vi "Balancing Controller.vi"(0 "Error In":errorcluster, 1 "steering indicator flag":i16, 5 "Trajectory In":refnum<data-value>, 6 "Balance In":refnum<data-value>, 9 "State Estimate In":refnum<data-value>, 10 "t":i32, 11 "Measurement In":refnum<data-value>, 12 "Indoor (RollRef)":bool=TRUE, 13 "Configuration":T1={"Accelerometer Bias"={"X (m/s)"=0.0, "Y (m/s)"=0.0, "Z (m/s)"=0.0}, "Gyroscope Bias"={"X (m/s)"=0.0, "Y (m/s)"=0.0, "Z (m/s)"=0.0}, "Steering Motor Gear Ratio"=611.0, "Steering Pully Gear Ratio"=1.0, "Steering Encoder CPR"=500.0, "Steering Motor Max RPM"=4000.0, "Wheelbase (m)"=1.12, "Fork Angle (rad)"=1.3, "Balancing Controller"={"Kp (/s)"=1.0, "Kd (1)"=1.0}, "Max Allowed Steering Angle (rad)"=0.7, "Task Periods"={"Emergency Stop (us)"=10000, "IMU (us)"=10000, "Steering Motor Encoder (us)"=10000, "State Estimator (us)"=10000, "Balancing Controller (us)"=10000, "GNSS (us)"=10000, "Logging (us)"=50000, "Drive Motor (us)"=100000, "Visualization (us)"=50000}, "Drive Motor Gear Ratio"=0.7, "lr"=0.4964, "lf"=0.5986, "lambda"=1.2217, "k1"=0.004472, "k2"=0.09678, "e1_max"=11.331, "Ad_t"=0.95971, "Bd_t"=0.01, "C_t"=2.20588, "D_t"=0.0, "Wheel radius"=0.311}) -> (3 "Input balancing":dbl, 4 "Error Out":errorcluster, 14 "Steering Angle Rate (rad/s)":dbl, 15 "Measurement Out":refnum<data-value>)   [LabVIEW 2021]
uses:
  State Estimator/State Estimate.ctl
  State Estimator/Measurements.ctl
  IMU/IMU Data.ctl
  Steering Motor Encoder/Steering Motor Encoder Data.ctl
  GNSS/GNSS Data.ctl
  Trajectory Control/Trajectory_Control.ctl
  Configuration/Configuration.ctl
  Logging/Log Level.ctl
panel:
  in  "Balancing Controller.Kd (1)":dbl=3.5
  in  "Balancing Controller.Kp (/s)":dbl=3.75
  out "disturbances ref":dbl(graph)
  out "Balance Out":refnum<data-value>
  out "Trajectory out":refnum<data-value>
  out "State Estimate Out":refnum<data-value>
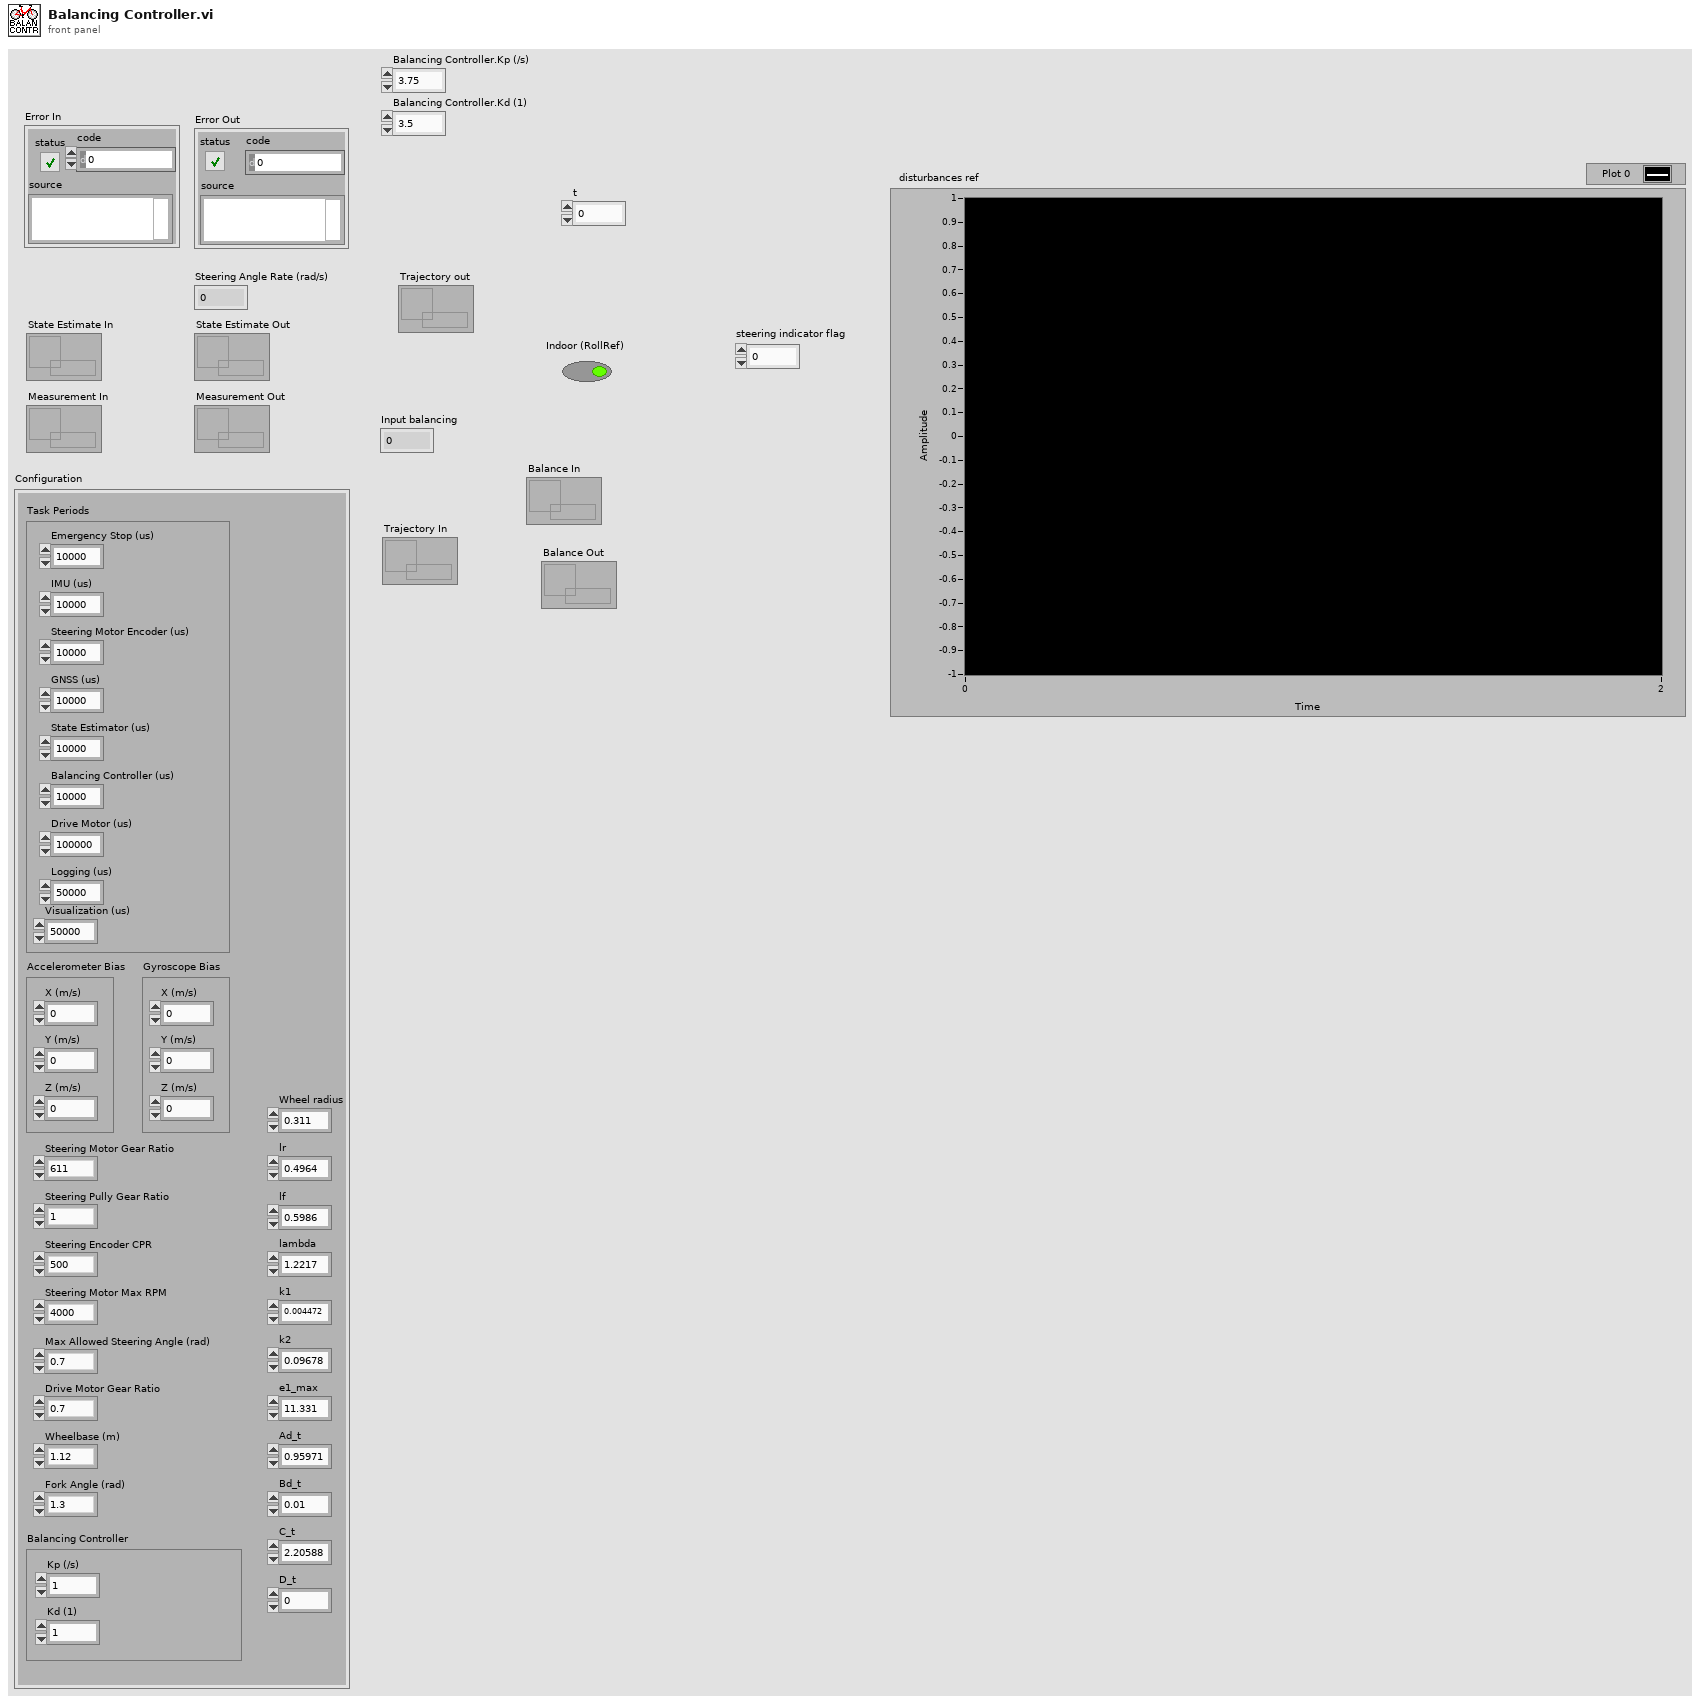
[diagram p1: front panel]
types:
  T1 = typedef "Configuration.ctl" = cluster{"Accelerometer Bias":cluster{"X (m/s)":dbl, "Y (m/s)":dbl, "Z (m/s)":dbl}, "Gyroscope Bias":cluster{"X (m/s)":dbl, "Y (m/s)":dbl, "Z (m/s)":dbl}, "Steering Motor Gear Ratio":dbl, "Steering Pully Gear Ratio":dbl, "Steering Encoder CPR":dbl, "Steering Motor Max RPM":dbl, "Wheelbase (m)":dbl, "Fork Angle (rad)":dbl, "Balancing Controller":cluster{"Kp (/s)":dbl, "Kd (1)":dbl}, "Max Allowed Steering Angle (rad)":dbl, "Task Periods":cluster{"Emergency Stop (us)":i64, "IMU (us)":i64, "Steering Motor Encoder (us)":i64, "State Estimator (us)":i64, "Balancing Controller (us)":i64, "GNSS (us)":i64, "Logging (us)":i64, "Drive Motor (us)":i64, "Visualization (us)":i64}, "Drive Motor Gear Ratio":dbl, "lr":dbl, "lf":dbl, "lambda":dbl, "k1":dbl, "k2":dbl, "e1_max":dbl, "Ad_t":dbl, "Bd_t":dbl, "C_t":dbl, "D_t":dbl, "Wheel radius":dbl}
  T2 = cluster{"Steering Angle Rate":dbl, "rollReference":dbl, "roll":dbl, "rollRate":dbl, "Kp":dbl, "Kd":dbl, "steering_flag":i32}
  T3 = typedef "Log Level.ctl" = enum16{"Error", "Warning", "Info"}
  T4 = typedef "Trajectory_Control.ctl" = cluster{"Rollref":dbl, "Closestpoint":dbl, "Error1":dbl, "Error2":dbl, "Dpsiref_cont":dbl, "Lateral_cont":dbl, "Heading_cont":dbl, "Reset_traj":dbl, "Iteration":dbl, "E1 limit":u32, "E2 limit":u32}
  T5 = typedef "State Estimate.ctl" = cluster{"X (m)":dbl, "Y (m)":dbl, "Psi (rad)":dbl, "Roll (rad)":dbl, "Roll Rate (rad/s)":dbl, "delta":dbl, "velocity":dbl, "Iterations":dbl}
  T6 = typedef "Measurements.ctl" = cluster{"IMU Data":T7, "Steering Motor Encoder Data":T8, "GNSS Data":T9}
  T7 = typedef "IMU Data.ctl" = cluster{"Gyroscope":cluster{"X (rad/s)":dbl, "Y (rad/s)":dbl, "Z (rad/s)":dbl}, "Accelerometer":cluster{"X (m/s^2)":dbl, "Y (m/s^2)":dbl, "Z (m/s^2)":dbl}, "Flag IMU":dbl}
  T8 = typedef "Steering Motor Encoder Data.ctl" = cluster{"Encoder Position (counts)":i32, "Steering Angle (rad)":dbl, "Steering Encoder Iteration":dbl}
  T9 = typedef "GNSS Data.ctl" = cluster{"Latitude (rad)":dbl, "Longitude (rad)":dbl, "Altitude (m)":dbl, "Speed (m/s)":dbl, "Heading (rad)":dbl, "Fix Quality":i32, "Number of Satellites":i32, "Latitude (deg)":dbl, "Longitude (deg)":dbl, "Flag GNSS":dbl}
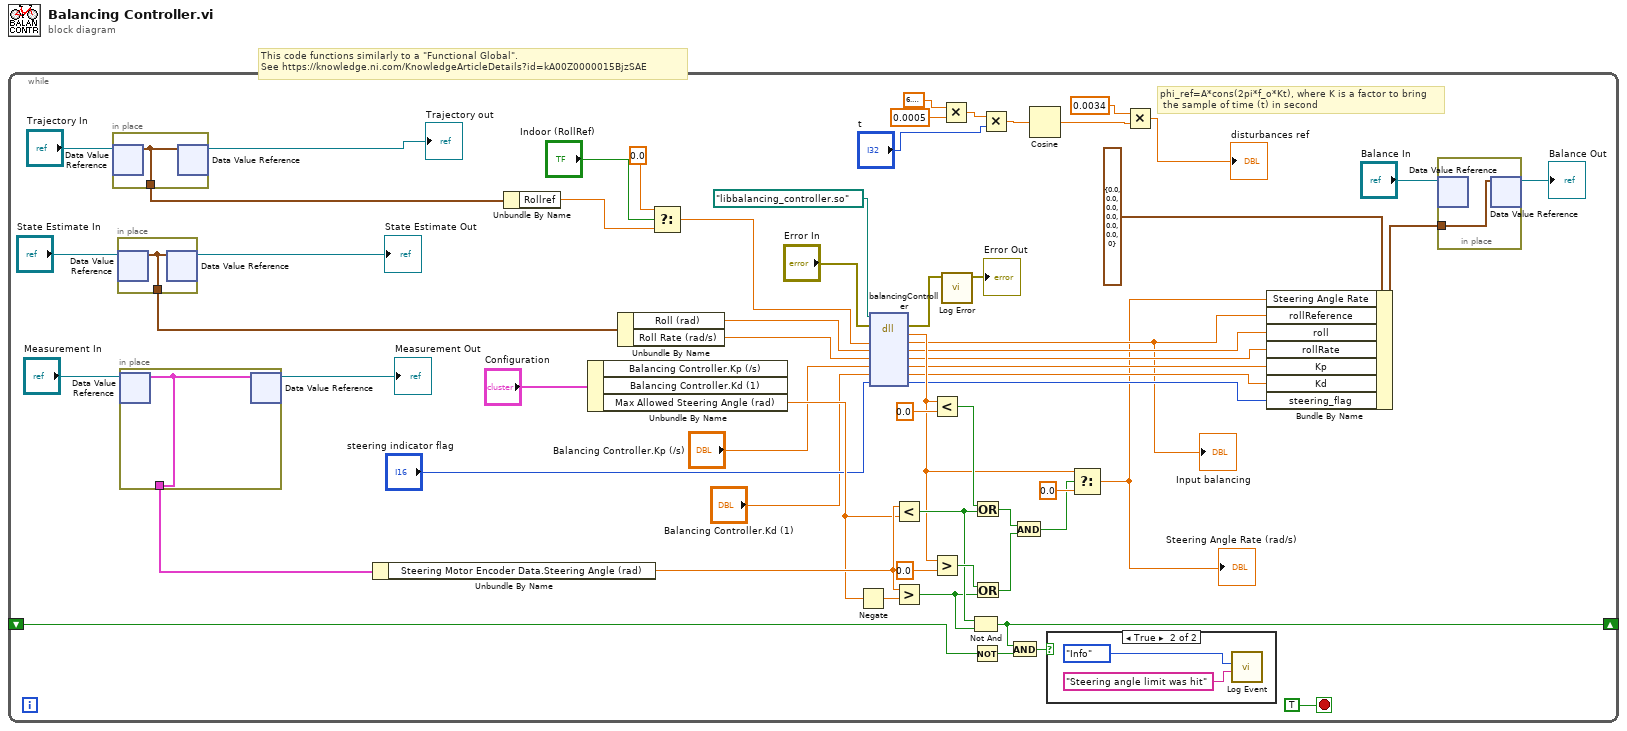
[diagram p0: block diagram]
diagram:
  # "This code functions similarly to a \"Functional Global\".\nSee https://knowledge.ni.com/KnowledgeArticleDetails?id=kA00Z0000015BjzSAE"
  n1 = while {
    shift-right: [w36] -> _
    shift-left: _ -> [w38]
    stop <- TRUE stop-if-true
    # "phi_ref=A*cons(2pi*f_o*Kt), where K is a factor to bring\n the sample of time (t) in second"
    n2 = in-place {
      in-place-border: [w63] -> w32
      n3 = in-place-dvr #1 ("Data Value Reference Read / Write Element")("Trajectory In") -> (w63:T4)  [unwired: 1 out]
      n4 = in-place-dvr #1(w63) -> (→"Trajectory out":refnum<data-value>)  [unwired: 1 out]
    }
    n5 = in-place {
      in-place-border: [w67] -> w57
      n6 = in-place-dvr #2("State Estimate In") -> (w67:T5)  [unwired: 1 out]
      n7 = in-place-dvr #2(w67) -> (→"State Estimate Out":refnum<data-value>)  [unwired: 1 out]
    }
    n8 = in-place {
      in-place-border: [w66] -> w54
      n9 = in-place-dvr #3("Measurement In") -> (w66:T6)  [unwired: 1 out]
      n10 = in-place-dvr #3(w66) -> (→"Measurement Out":refnum<data-value>)  [unwired: 1 out]
    }
    n11 = Unbundle By Name(w54) -> ("Steering Motor Encoder Data.Steering Angle (rad)"=w44:dbl)
    n12 = Unbundle By Name(w32) -> ("Rollref"=w5:dbl)
    n13 = Unbundle By Name("Configuration") -> ("Max Allowed Steering Angle (rad)"=w43:dbl)  [unwired: 2 out]
    n14 = Unbundle By Name(w57) -> ("Roll (rad)"=w29:dbl, "Roll Rate (rad/s)"=w28:dbl)
    n15 = Select(t=0.0 ("rollReference"), s="Indoor (RollRef)", f=w5) -> (s? t:f=w4:dbl)
    n16 = Negate(x=w43) -> (-x=w45:dbl)
    n17 = dll-call lib="?" fn="balancingController"(path in=path "libbalancing_controller.so", error in="Error In", "rollReference"=w4, "roll"=w29, "rollRate"=w28, "Kp"="Balancing Controller.Kp (/s)", "Kd"="Balancing Controller.Kd (1)", "steering_flag"="steering indicator flag") -> (error out=w41:errorcluster, "Steering Angle Rate"=w26:dbl, "rollReference"=w2:dbl, "roll"=w25:dbl, "rollRate"=w24:dbl, "Kp"=w23:dbl, "Kd"=w22:dbl, "steering_flag"=w21:i32)  [unwired: 1 in, 1 out]
    "Input balancing" <- w2
    n18 = Less?(x=w44, y=w43) -> (x < y?=w35:bool)
    n19 = Greater?(x=w44, y=w45) -> (0:w34:bool)
    n20 = Less?(x=w26, y=0.0) -> (x < y?=w51:bool)
    n21 = Greater?(x=w26, y=0.0) -> (0:w48:bool)
    n22 = Multiply(x=6.283185307179586, y=0.0005) -> (x*y=w18:dbl)
    n23 = call "Log Error.vi"("Error In"=w41) -> ("Error Out"=→"Error Out":errorcluster)  [unwired: 10 in]
    n24 = Not And(1:w34, 2:w35) -> (0:w36:bool)
    n25 = Not(x=w38) -> (.not. x?=w39:bool)
    n26 = Or(x=w51, y=w35) -> (x .or. y?=w50:bool)
    n27 = Or(x=w48, y=w34) -> (x .or. y?=w47:bool)
    n28 = Multiply(x=w18, y="t") -> (x*y=w16:dbl)
    n29 = And(x=w36, y=w39) -> (x .and. y?=w37:bool)
    n30 = And(x=w50, y=w47) -> (x .and. y?=w46:bool)
    n31 = Cosine(x=w16) -> (cos(x)=w15:dbl)
    n32 = case shown="True" w37 {
      frame False {
      }
      frame True {
        n33 = call "Log Event.vi"("Message"="Steering angle limit was hit", "Log Level"=Log_Level."Info") -> ()  [unwired: 9 in, 1 out]
      }
    }
    n34 = Select(t=w26, s=w46, f=0.0) -> (s? t:f=w1:dbl)
    "Steering Angle Rate (rad/s)" <- w1
    n35 = Multiply(x=0.0034, y=w15) -> (x*y=→"disturbances ref":dbl)
    n36 = Bundle By Name(cluster=T2 {"Steering Angle Rate"=0.0, "rollReference"=0.0, "roll"=0.0, "rollRate"=0.0, "Kp"=0.0, "Kd"=0.0, "steering_flag"=0}, "Steering Angle Rate"=w1, "rollReference"=w2, "roll"=w25, "rollRate"=w24, "Kp"=w23, "Kd"=w22, "steering_flag"=w21) -> (w12:T2)
    n37 = in-place {
      in-place-border: w12 -> [w62]
      n38 = in-place-dvr #4("Balance In") -> ()  [unwired: 2 out]
      n39 = in-place-dvr #4(w62) -> (→"Balance Out":refnum<data-value>)  [unwired: 1 out]
    }
  }
